vi "Ex2Task1_Main.vi"() -> ()   [LabVIEW 2014, in "Singh_3rd_Ex2Task1_12-6-16.lvrbt"]
uses:
  Singh_3rd_Ex2Task1_12-6-16.lvrbt
  <vilib>/NXT/Dual Mode Library/Display/drawText.vi
panel:
  out "Result":dbl
  out "A+B":dbl
  in  "B":dbl
  in  "A":dbl
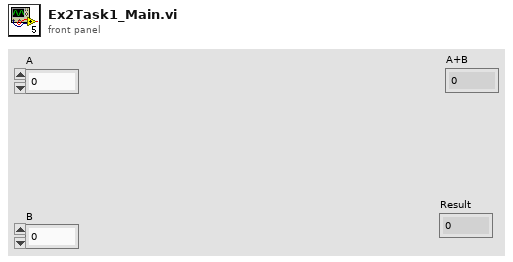
[diagram p1: front panel]
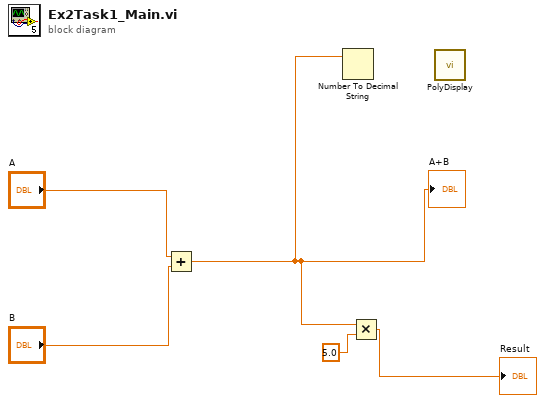
[diagram p0: block diagram]
diagram:
  n1 = Add(x="A", y="B") -> (x+y=w1:dbl)
  "A+B" <- w1
  n2 = Number To Decimal String(number=w1) -> ()  [unwired: 1 in, 1 out]
  n3 = Multiply(x=w1, y=5.0) -> (x*y=→"Result":dbl)
  n4 = call-poly <vilib>:"PolyDisplay.vi"() -> ()  [unwired: 4 in, 1 out]
